vi "labview_vhdl.vi"   [LabVIEW 2015]
uses:
  <vilib>/rvi/IPIntegrationNode/IPINode_Xnode/niFpgaIPINode.xnode
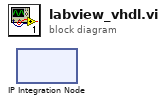
[diagram p0: block diagram]
diagram:
  n1 = xnode "IP Integration Node"() -> ()
